vi "Advance past whitespace.vi"(4 "Past Colon":bool, 6 "Past Comma":bool, 7 "JSON":string, 9 "Offset":i32, 11 "Parser State in":T1=enum."Leading Whitespace") -> (1 "Offset of first non-whitespace":i32, 3 "Parser State":T1)   [LabVIEW 2013, in "JSONtext.lvlib"]
uses:
  JSONtext.lvlib
  Parsing State.ctl
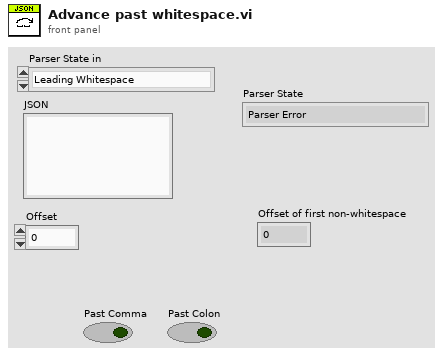
[diagram p1: front panel]
types:
  T1 = typedef "JSONtext.lvlib/Parsing State.ctl" = enum16{"Parser Error", "Object", "Array", "String", "Number/Other", "Leading Whitespace", "Object end", "Array end", "Value end"}
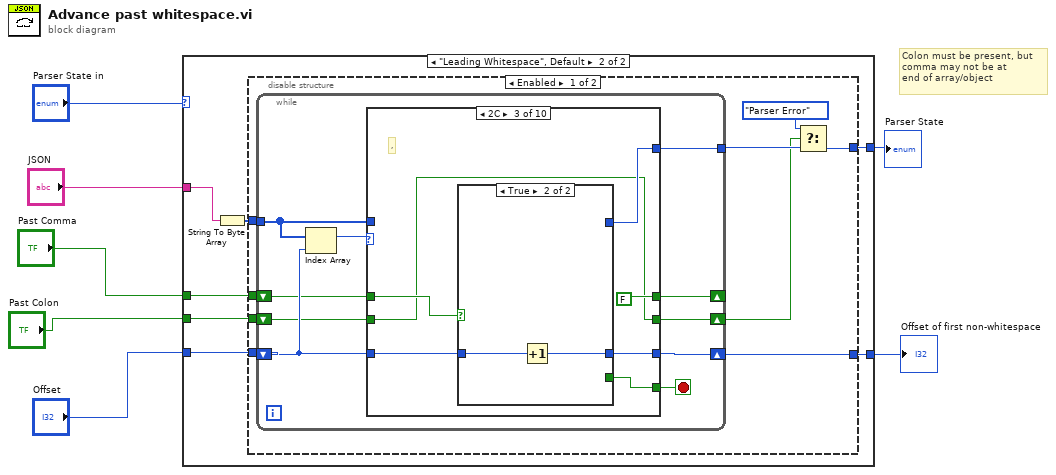
[diagram p0: block diagram]
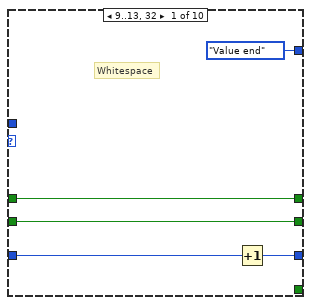
[diagram p3: hidden frame]
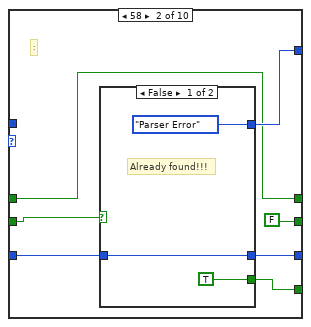
[diagram p4: hidden frame]
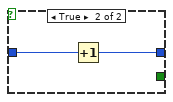
[diagram p5: hidden frame]
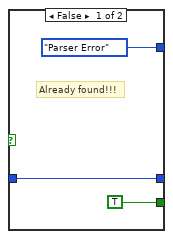
[diagram p6: hidden frame]
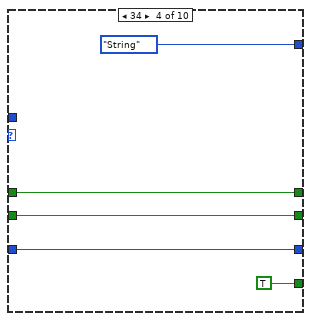
[diagram p7: hidden frame]
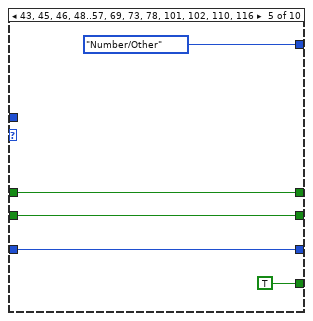
[diagram p8: hidden frame]
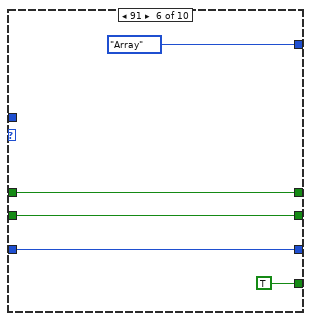
[diagram p9: hidden frame]
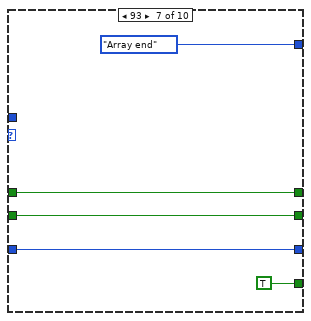
[diagram p10: hidden frame]
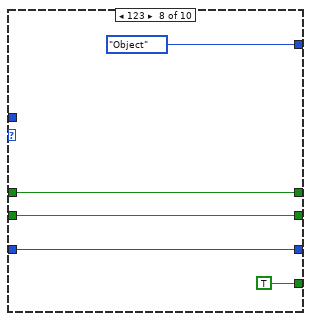
[diagram p11: hidden frame]
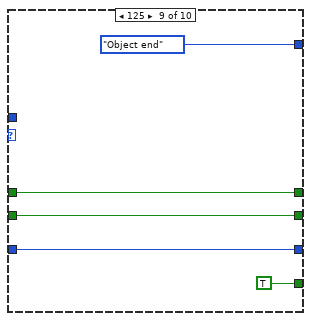
[diagram p12: hidden frame]
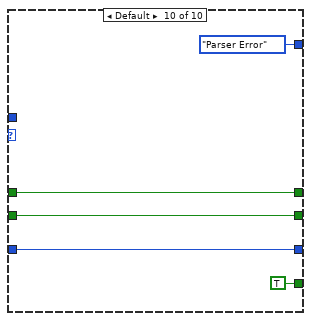
[diagram p13: hidden frame]
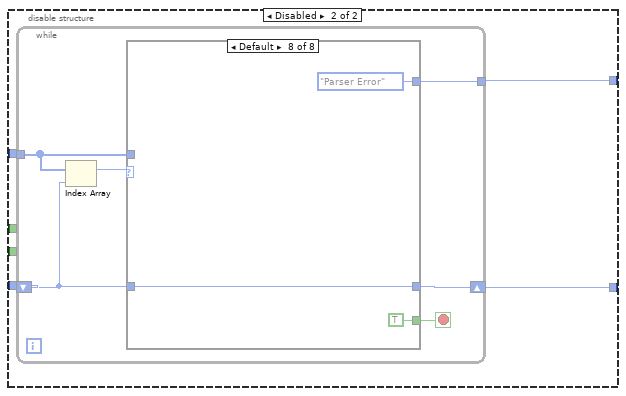
[diagram p14: hidden frame]
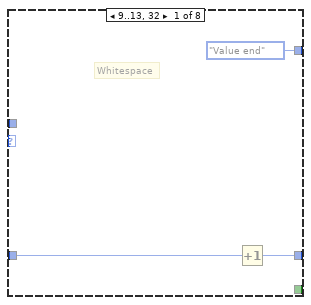
[diagram p15: hidden frame]
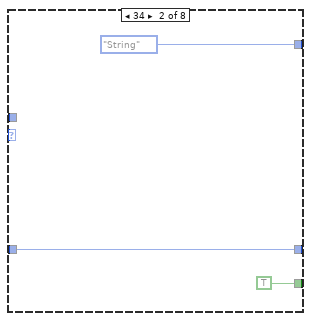
[diagram p16: hidden frame]
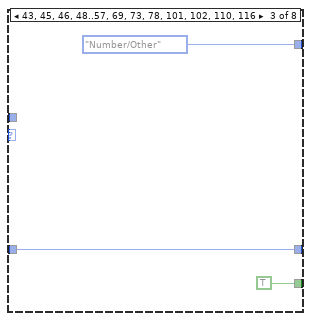
[diagram p17: hidden frame]
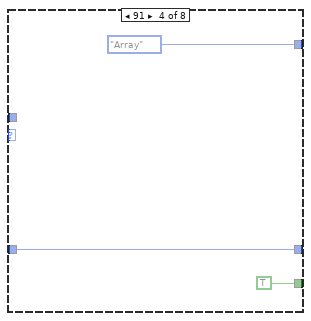
[diagram p18: hidden frame]
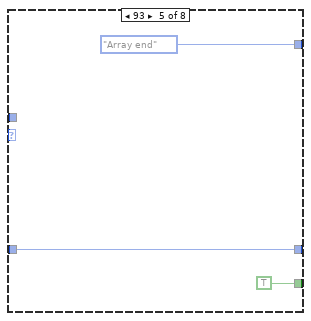
[diagram p19: hidden frame]
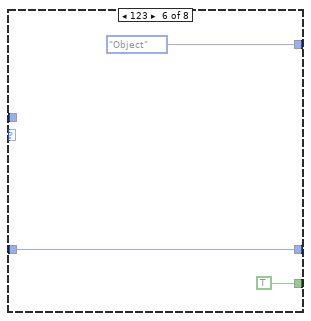
[diagram p20: hidden frame]
diagram:
  # "Colon must be present, but\ncomma may not be at\nend of array/object"
  n1 = case shown="\"Leading Whitespace\", Default" "Parser State in" {
    selector: "Parser State in" -> [w9 _]
    tunnel: [w9 w16] -> w7
    tunnel: [w8 w15] -> w6
    tunnel: "Offset" -> [w8 w14]
    tunnel: "JSON" -> [_ w13]
    tunnel: "Past Comma" -> [_ w12]
    tunnel: "Past Colon" -> [_ w11]
    frame "Parser Error" {
    }
    frame "Leading Whitespace", Default {
      n2 = String To Byte Array(string=w13) -> (unsigned byte array=w10:u8[])
      n3 = disable-structure shown="Enabled" {
        disable-tunnel: [w19 w103] -> w16
        disable-tunnel: [w24 w102] -> w15
        disable-tunnel: w14 -> [w23 w101]
        disable-tunnel: w12 -> [w22 _]
        disable-tunnel: w11 -> [w21 _]
        disable-tunnel: w10 -> [w20 w100]
        frame Enabled {
          n4 = while {
            tunnel: w20 -> [w34]
            shift-right: [w30] -> w24
            shift-left: w23 -> [w31]
            tunnel: [w33] -> w25
            shift-right: [w29] -> _
            shift-left: w22 -> [w28]
            shift-right: [w26] -> w17
            shift-left: w21 -> [w27]
            stop <- w32 stop-if-true
            n5 = Index Array(array=w34, index=w31) -> (element=w35:u8)
            n6 = case shown="2C" w35 {
              tunnel: w34 -> [_ _ _ _ _ _ _ _ _ _]
              tunnel: [Parsing_State."Value end" w45 w57 Parsing_State."String" Parsing_State."Number/Other" Parsing_State."Array" Parsing_State."Array end" Parsing_State."Object" Parsing_State."Object end" Parsing_State."Parser Error"] -> w33
              tunnel: [_ w44 w56 TRUE TRUE TRUE TRUE TRUE TRUE TRUE] -> w32
              tunnel: w31 -> [w40 w47 w59 w67 w72 w77 w82 w87 w92 w99]
              tunnel: [w39 w46 w58 w67 w72 w77 w82 w87 w92 w99] -> w30
              tunnel: [w37 w41 FALSE ("Allow Comma") w66 w71 w76 w81 w86 w91 w96] -> w29
              tunnel: w28 -> [w37 w41 w55 w66 w71 w76 w81 w86 w91 w96]
              tunnel: [w36 FALSE ("Allow Comma") w53 w65 w70 w75 w80 w85 w90 w95] -> w26
              tunnel: w27 -> [w36 w43 w53 w65 w70 w75 w80 w85 w90 w95]
              frame 9..13, 32 {
                # "Whitespace"
                n7 = Increment(x=w40) -> (x+1=w39:i32)
              }
              frame 58 {
                # ":"
                n8 = case shown="False" w43 {
                  tunnel: w47 -> [w49 w52]
                  tunnel: [w49 w51] -> w46
                  tunnel: [Parsing_State."Parser Error" _] -> w45
                  tunnel: [TRUE _] -> w44
                  frame False {
                    # "Already found!!!"
                  }
                  frame True {
                    n9 = Increment(x=w52) -> (x+1=w51:i32)
                  }
                }
              }
              frame 44 {
                # ","
                n10 = case shown="True" w55 {
                  tunnel: w59 -> [w61 w64]
                  tunnel: [w61 w63] -> w58
                  tunnel: [Parsing_State."Parser Error" _] -> w57
                  tunnel: [TRUE _] -> w56
                  frame False {
                    # "Already found!!!"
                  }
                  frame True {
                    n11 = Increment(x=w64) -> (x+1=w63:i32)
                  }
                }
              }
              frame 34 {
              }
              frame 43, 45, 46, 48..57, 69, 73, 78, 101, 102, 110, 116 {
              }
              frame 91 {
              }
              frame 93 {
              }
              frame 123 {
              }
              frame 125 {
              }
              frame Default {
              }
            }
          }
          n12 = Select(t=Parsing_State."Parser Error", s=w17, f=w25) -> (s? t:f=w19:T1)
        }
        frame Disabled {
          n13 = while {
            tunnel: w100 -> [w108]
            shift-right: [w104] -> w102
            shift-left: w101 -> [w105]
            tunnel: [w107] -> w103
            stop <- w106 stop-if-true
            n14 = Index Array(array=w108, index=w105) -> (element=w109:u8)
            n15 = case shown="Default" w109 {
              tunnel: w108 -> [_ _ _ _ _ _ _ _]
              tunnel: [Parsing_State."Value end" Parsing_State."String" Parsing_State."Number/Other" Parsing_State."Array" Parsing_State."Array end" Parsing_State."Object" Parsing_State."Object end" Parsing_State."Parser Error"] -> w107
              tunnel: [_ TRUE TRUE TRUE TRUE TRUE TRUE TRUE] -> w106
              tunnel: w105 -> [w112 w113 w116 w119 w122 w125 w128 w133]
              tunnel: [w111 w113 w116 w119 w122 w125 w128 w133] -> w104
              frame 9..13, 32 {
                # "Whitespace"
                n16 = Increment(x=w112) -> (x+1=w111:i32)
              }
              frame 34 {
              }
              frame 43, 45, 46, 48..57, 69, 73, 78, 101, 102, 110, 116 {
              }
              frame 91 {
              }
              frame 93 {
              }
              frame 123 {
              }
              frame 125 {
              }
              frame Default {
              }
            }
          }
        }
      }
    }
  }
  "Parser State" <- w7
  "Offset of first non-whitespace" <- w6
